vi "Scaled XOR Eval.vi"(11 "Neural Network Out":refnum<class "Neural Network.lvclass">) -> (2 "Output 1":refnum<class "3D Plot Datatype.lvclass">[](array[class]), 3 "Output 0":refnum<class "3D Plot Datatype.lvclass">[](array[class]))   [LabVIEW 2015]
uses:
  Neural Network/Neural Network.lvclass
  <vilib>/Math Plots/3D Math Plots/3D Surface/3D Surface Datatype/3D Surface Datatype.lvclass
  <vilib>/Math Plots/3D Math Plots/3D Surface/3D Surface Datatype/Public/Plot Helper (Vector).vi
  <vilib>/Math Plots/3D Math Plots/3D Plot/3D Plot Datatype/3D Plot Datatype.lvclass
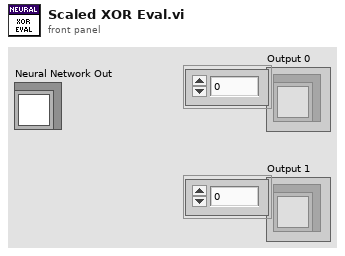
[diagram p1: front panel]
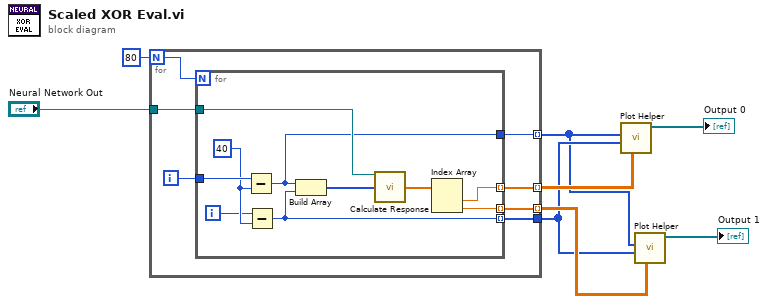
[diagram p0: block diagram]
diagram:
  n1 = for {
    N: 80 -> [w15]
    tunnel: "Neural Network Out" -> [w13]
    tunnel: [w12] -> w1 mode=indexing
    tunnel: [w11] -> w2
    tunnel: [w10] -> w8 mode=indexing
    tunnel: [w9] -> w3 mode=indexing
    i -> [w14]
    n2 = for {
      N: w15 -> [_]
      tunnel: w14 -> [w25]
      tunnel: w13 -> [w22]
      tunnel: [w21] -> w12
      tunnel: [w20] -> w11 mode=indexing
      tunnel: [w19] -> w10 mode=indexing
      tunnel: [w18] -> w9 mode=indexing
      i -> [w23]
      w24 = 40 ("y")
      n3 = Subtract(x=w25, y=w24) -> (x-y=w21:i32)
      n4 = Subtract(x=w23, y=w24) -> (x-y=w20:i32)
      n5 = Build Array(w21, w20) -> (w16:i32[])
      n6 = call "Calculate Response.vi"("Neural Network In"=w22, "Inputs"=w16) -> ("Outputs"=w17:dbl[])  [unwired: 11 in, 2 out]
      n7 = Index Array(array=w17) -> (element #1=w19:dbl, element #2=w18:dbl)  [unwired: 2 in]
    }
  }
  n8 = call-poly <vilib>:"Plot Helper.vi"("z matrix"=w8, "y vector"=w2, "x vector"=w1) -> ("3D Plot lvclass Array out"=→"Output 0":refnum<class "3D Plot Datatype.lvclass">[])  [unwired: 3 in, 5 out]
  n9 = call-poly <vilib>:"Plot Helper.vi"("z matrix"=w3, "y vector"=w2, "x vector"=w1) -> ("3D Plot lvclass Array out"=→"Output 1":refnum<class "3D Plot Datatype.lvclass">[])  [unwired: 3 in, 5 out]
